vi "Measurement Logic.vi"() -> ()   [LabVIEW 2021, in "Scalar Efficiency And Load Regulation_PMIC.lvlib"]
uses:
  Scalar Efficiency And Load Regulation_PMIC.lvlib
  Measurement Configuration.ctl
  Measurement Results.ctl
  <vilib>/Plug-In SDKs/Measurements/Measure Call Context/Measure Call Context.lvclass
  <instrlib>/niDCPower/nidcpower.llb/niDCPower Sense.ctl
  <instrlib>/niDCPower/nidcpower.llb/niDCPower Source Mode.ctl
  <instrlib>/niDCPower/nidcpower.llb/niDCPower Wait For Event - Event.ctl
  <instrlib>/niDCPower/nidcpower.llb/niDCPower Output Function.ctl
  <instrlib>/niDCPower/nidcpower.llb/niDCPower Get Channel Name From String.vi
  <instrlib>/niDCPower/nidcpower.llb/niDCPower Configure Digital Edge Source Trigger With Channels.vi
  <instrlib>/niDCPower/nidcpower.llb/niDCPower Configure Digital Edge Measure Trigger With Channels.vi
panel:
  out "measure call context out":refnum<class "Measure Call Context.lvclass">
  in  "measure call context in":refnum<class "Measure Call Context.lvclass">
  out "measurement results":T1
  in  "measurement configuration":T2={"Mode of operation"=enum."Perform measurement", "DUT setup time"=1.0, "Source delay"=0.005, "Aperture time"=0.005, "Nominal output voltage"=3.3, "Source resource name"="", "Source sense"=1009, "Source current limit"=25.0, "Source maximum power"=300.0, "Load resource name"="", "Load sense"=1009, "Load voltage limit range"=6.0, "Source Voltage"=0.0, "Load Current"=0.0} {"Load sense" items=["Local"=1008, "Remote"=1009]; "Source sense" items=["Local"=1008, "Remote"=1009]}
  out "error out":errorcluster
  in  "error in":errorcluster
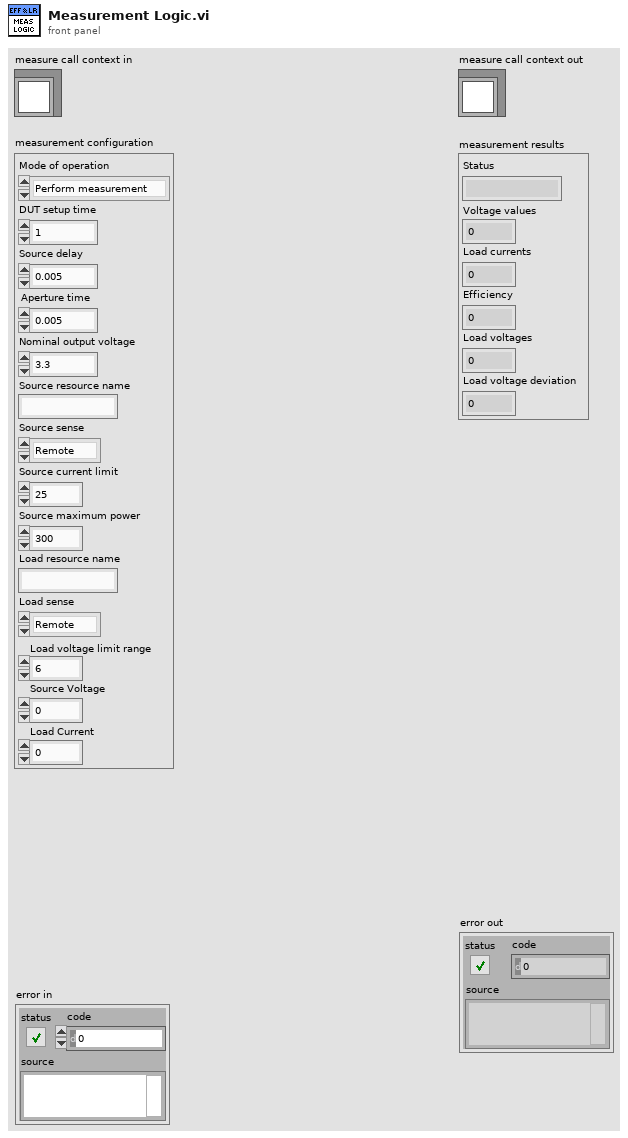
[diagram p1: front panel]
types:
  T1 = typedef "Scalar Efficiency And Load Regulation_PMIC.lvlib/Measurement Results.ctl" = cluster{"Status":string, "Voltage values":dbl, "Load currents":dbl, "Efficiency":dbl, "Load voltages":dbl, "Load voltage deviation":dbl}
  T2 = typedef "Scalar Efficiency And Load Regulation_PMIC.lvlib/Measurement Configuration.ctl" = cluster{"Mode of operation":enum32{"Power on the DUT", "Perform measurement", "Power off the DUT"}, "DUT setup time":dbl, "Source delay":dbl, "Aperture time":dbl, "Nominal output voltage":dbl, "Source resource name":string, "Source sense":i32, "Source current limit":dbl, "Source maximum power":dbl, "Load resource name":string, "Load sense":i32, "Load voltage limit range":dbl, "Source Voltage":dbl, "Load Current":dbl}
  T3 = cluster{"Voltage values":dbl, "Source out":refnum<k15>, "Source channel name":string, "Load out":refnum<k15>, "Load channel name":string, "Current values":dbl[], "Load sweep points":i32, "Source terminal name":string, "Measure terminal name":string, "Measurement Results":T1, "Source sequence name":string}
  T4 = enum32{"Power on the DUT", "Perform measurement", "Power off the DUT"}
  T5 = typedef "niDCPower Wait For Event - Event.ctl" = i32
  T6 = typedef "niDCPower Source Mode.ctl" = i32
  T7 = typedef "niDCPower Sense.ctl" = i32
  T8 = typedef "niDCPower Output Function.ctl" = i32
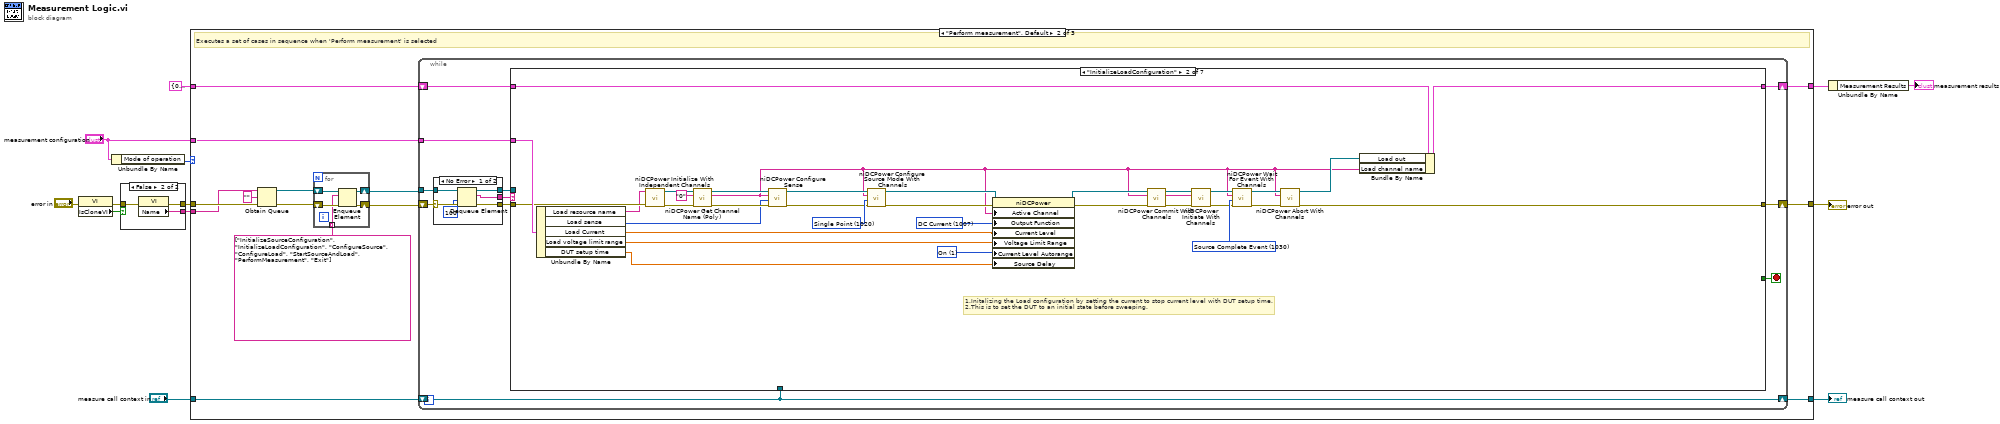
[diagram p0: block diagram]
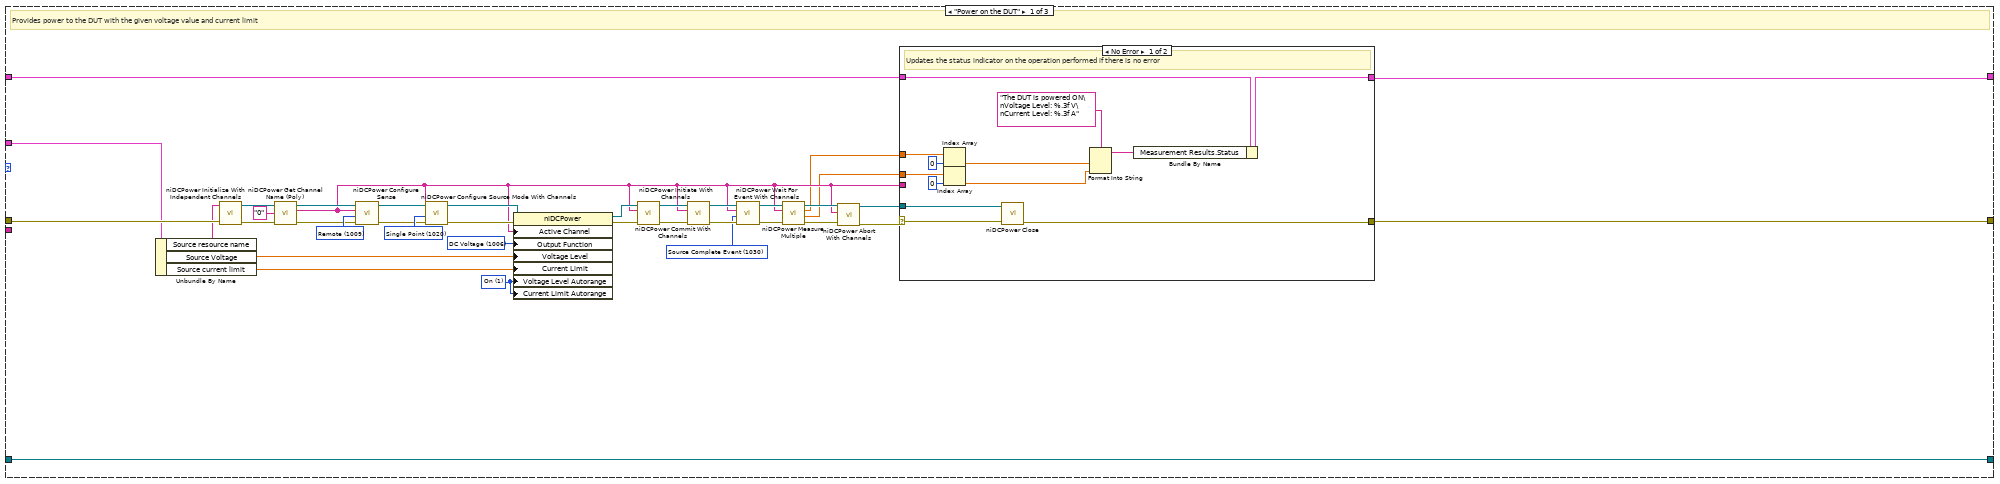
[diagram p2: hidden frame]
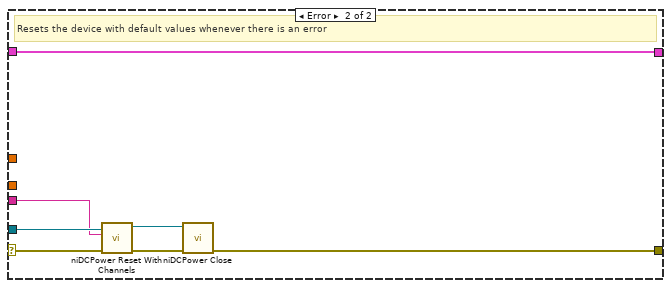
[diagram p3: hidden frame]
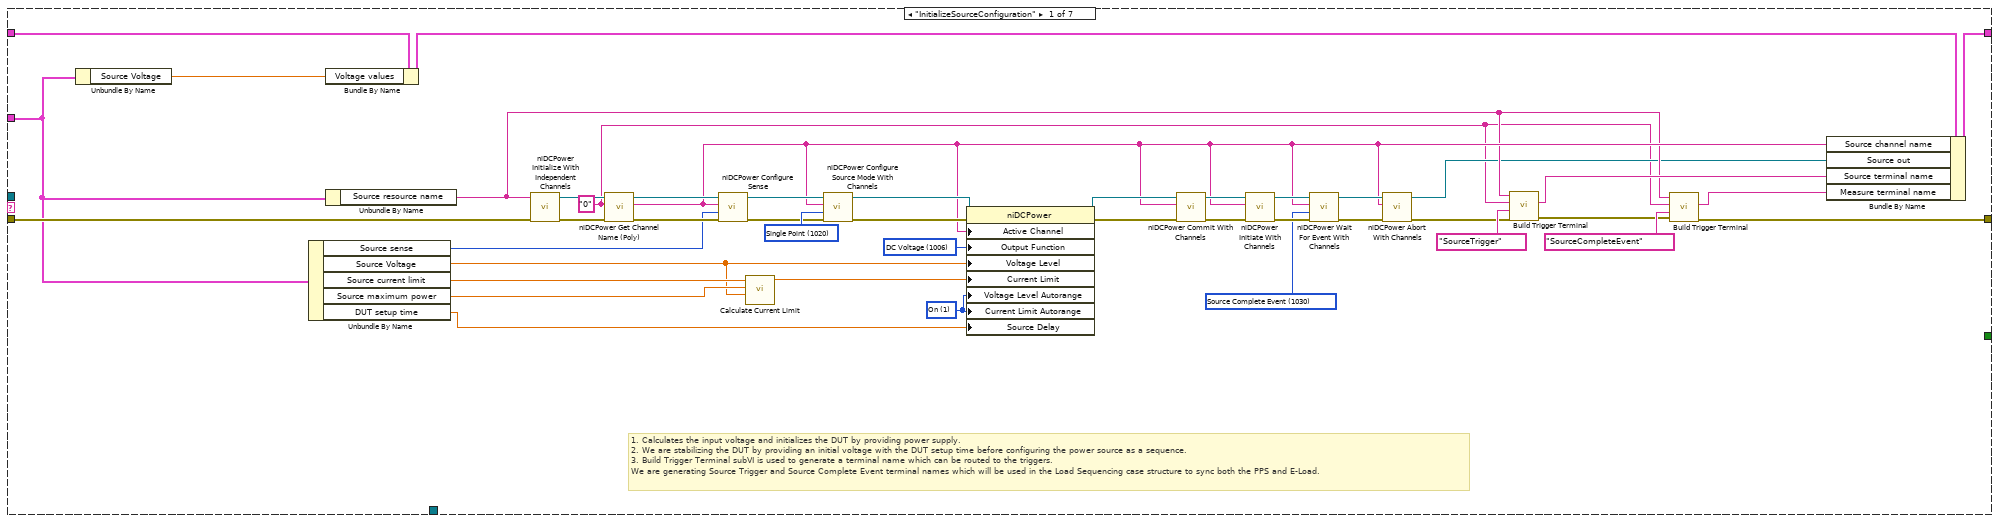
[diagram p4: hidden frame]
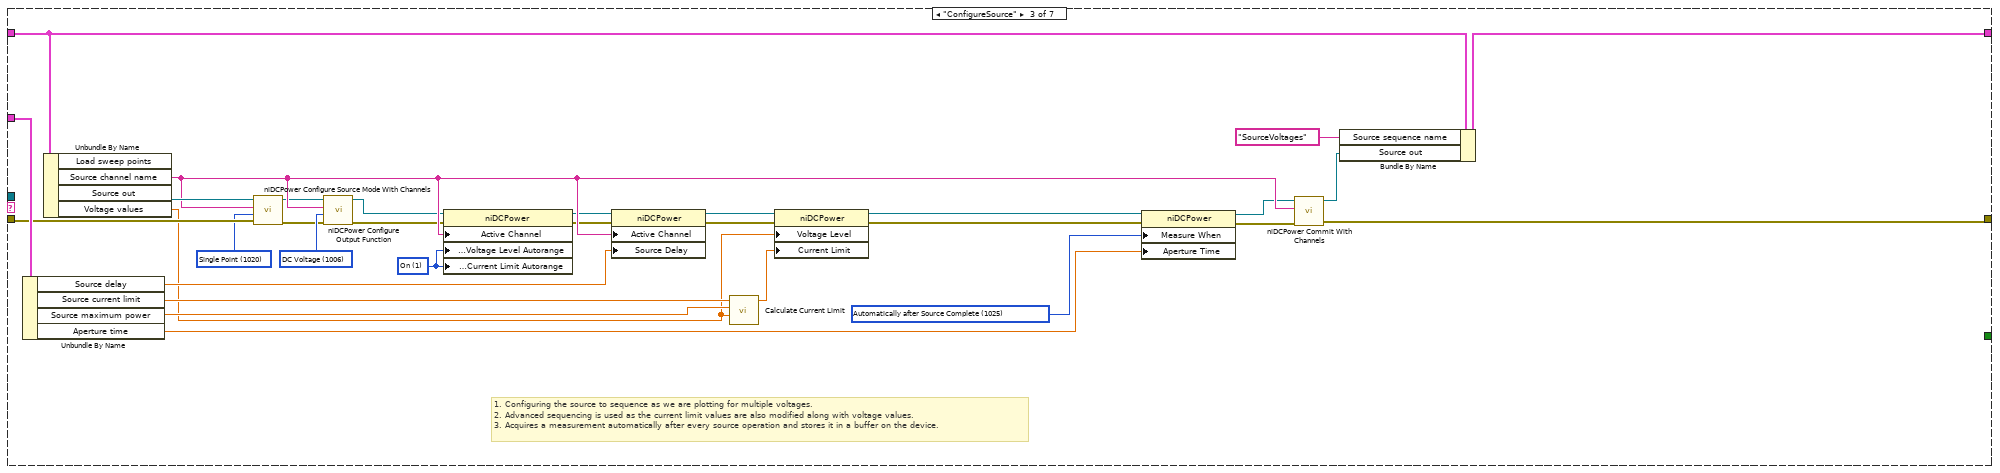
[diagram p5: hidden frame]
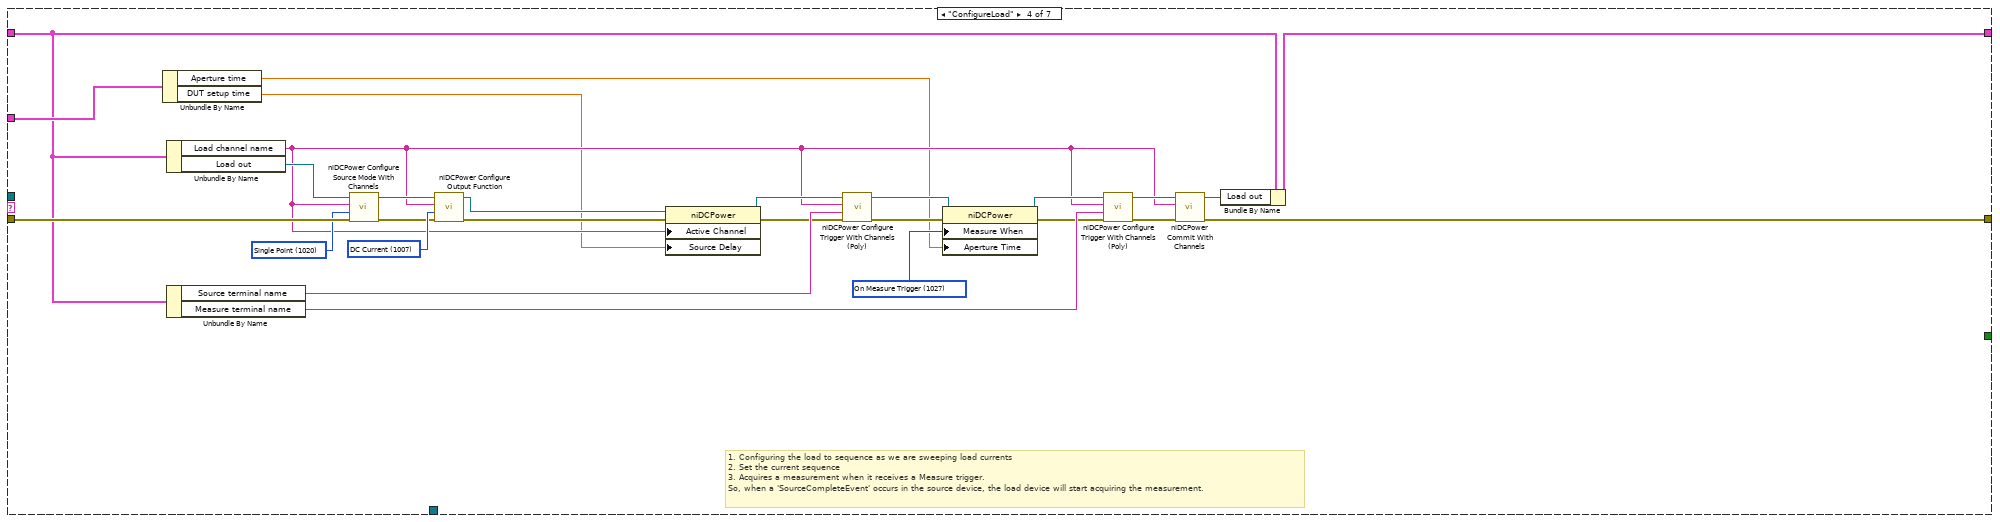
[diagram p6: hidden frame]
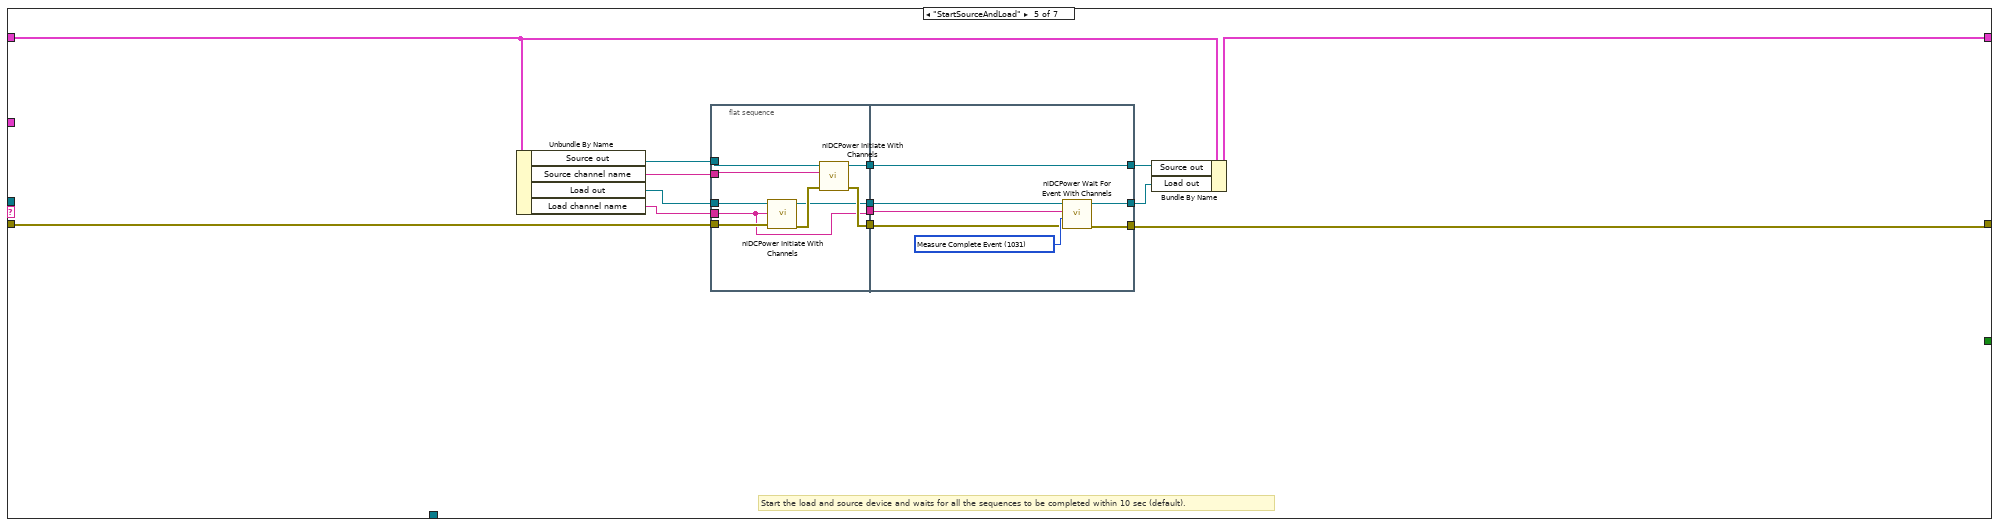
[diagram p7: hidden frame]
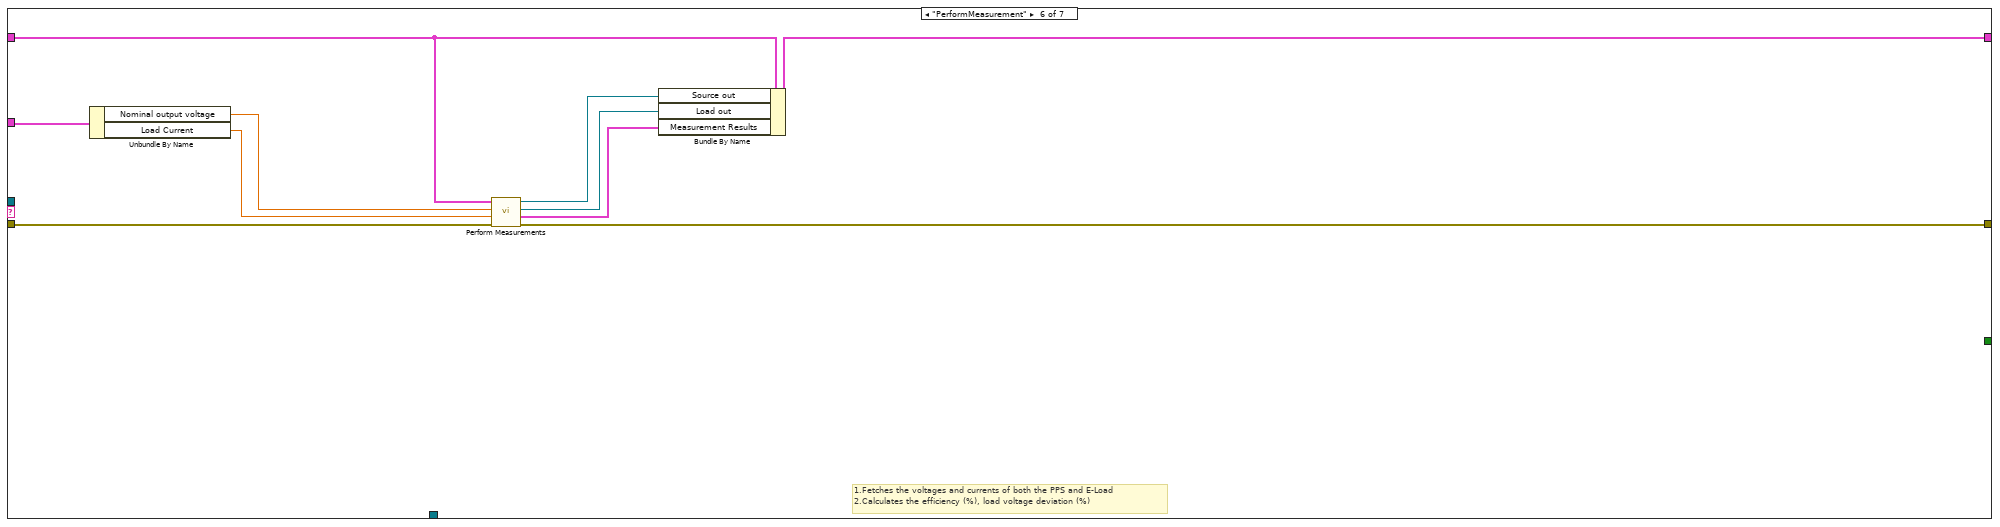
[diagram p8: hidden frame]
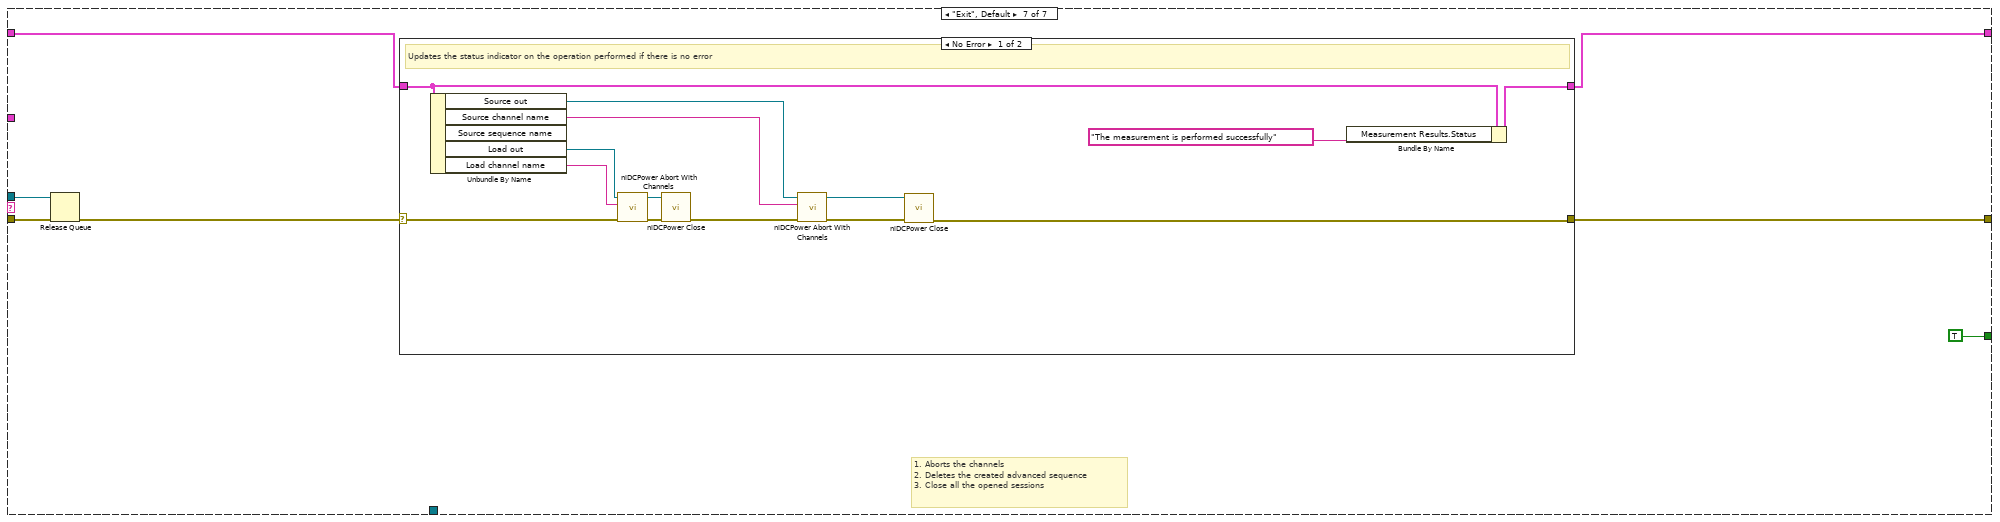
[diagram p9: hidden frame]
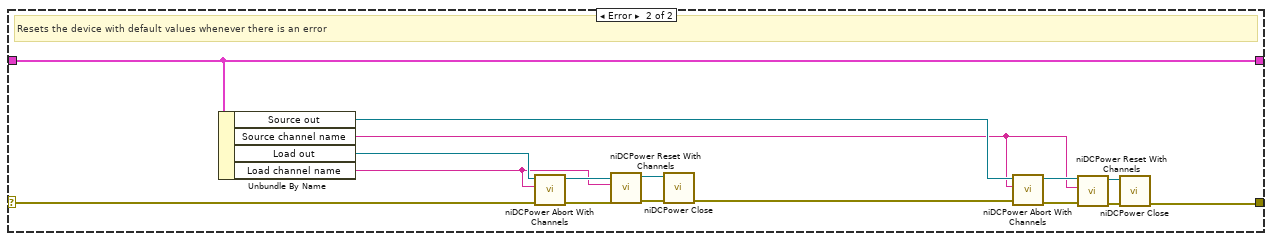
[diagram p10: hidden frame]
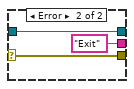
[diagram p11: hidden frame]
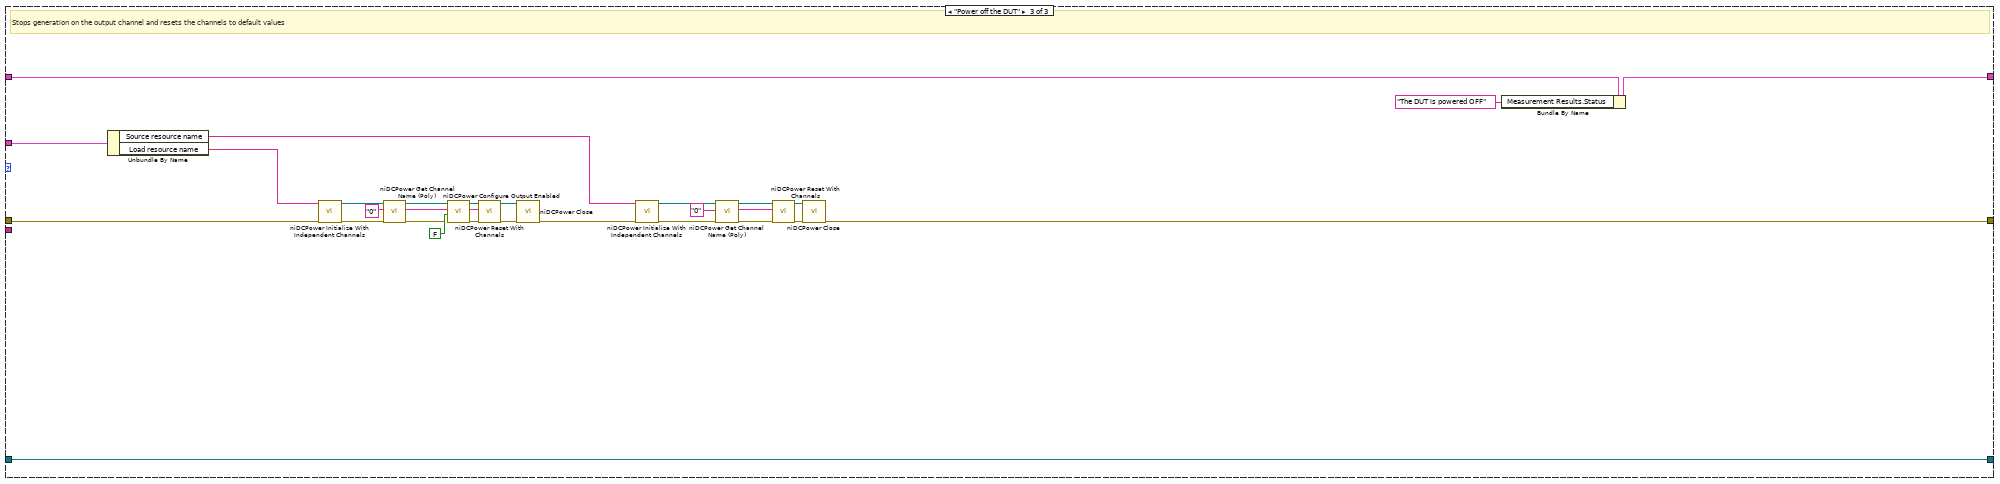
[diagram p12: hidden frame]
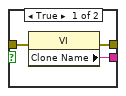
[diagram p13: hidden frame]
diagram:
  n1 = property class="VI"(error in="error in") -> (error out=w12:errorcluster, "IsCloneVI"=w13:bool)  [unwired: 1 in, 1 out]
  n2 = Unbundle By Name("measurement configuration") -> ("Mode of operation"=w5:T4)
  n3 = case shown="False" w13 {
    tunnel: [w16 w19] -> w7
    tunnel: [w15 w18] -> w6
    tunnel: w12 -> [w14 w17]
    frame True {
      n4 = property class="VI"(error in=w14) -> (error out=w16:errorcluster, "Clone Name"=w15:string)  [unwired: 1 in, 1 out]
    }
    frame False {
      n5 = property class="VI"(error in=w17) -> (error out=w19:errorcluster, "Name"=w18:string)  [unwired: 1 in, 1 out]
    }
  }
  n6 = case shown="\"Perform measurement\", Default" w5 {
    tunnel: [w21 w77 w344] -> w1
    tunnel: w7 -> [w37 w87 w343]
    tunnel: w6 -> [_ w86 _]
    tunnel: "measurement configuration" -> [w30 w83 w331]
    tunnel: [w22 w78 w327] -> w2
    tunnel: T3 {"Voltage values"=0.0, "Source out"="", "Source channel name"="", "Load out"="", "Load channel name"="", "Current values"=[], "Load sweep points"=0, "Source terminal name"="", "Measure terminal name"="", "Measurement Results"={"Status"="", "Voltage values"=0.0, "Load currents"=0.0, "Efficiency"=0.0, "Load voltages"=0.0, "Load voltage deviation"=0.0}, "Source sequence name"=""} -> [w23 w82 w329]
    tunnel: "measure call context in" -> [w20 w80 w330]
    tunnel: [w20 w79 w330] -> w3
    frame "Power on the DUT" {
      w40 = 1 items=["Off", "On"] ("Source:DC Voltage:Voltage Level Autorange")
      w41 = T5 1030 items=["Source Complete Event"=1030, "Measure Complete Event"=1031, "Sequence Iteration Complete Event"=1032, "Sequence Engine Done Event"=1033, "Pulse Complete Event"=1051, "Ready For Pulse Trigger Event"=1052] ("event")
      w52 = T6 1020 items=["Single Point"=1020, "Sequence"=1021] ("source mode")
      w47 = 1006 items=["DC Voltage"=1006, "DC Current"=1007, "Pulse Voltage"=1049, "Pulse Current"=1050] ("Source:Output Function")
      w42 = T7 1009 items=["Local"=1008, "Remote"=1009] ("sense")
      # "Provides power to the DUT with the given voltage value and current limit"
      n7 = Unbundle By Name(w30) -> ("Source resource name"=w34:string, "Source Voltage"=w29:dbl, "Source current limit"=w35:dbl)
      n8 = call <instrlib>:"niDCPower Initialize With Independent Channels.vi"("error in (no error)"=w37, "resource name"=w34) -> ("error out"=w39:errorcluster, "instrument handle out"=w43:refnum<k15>)  [unwired: 8 in]
      n9 = call-poly <instrlib>:"niDCPower Get Channel Name (Poly).vi"("index"="0", "instrument handle"=w43) -> ("name"=w26:string, "instrument handle out"=w38:refnum<k15>)  [unwired: 7 in, 1 out]
      n10 = call <instrlib>:"niDCPower Configure Sense.vi"("error in (no error)"=w39, "sense"=w42, "channel name"=w26, "instrument handle"=w38) -> ("error out"=w50:errorcluster, "instrument handle out"=w48:refnum<k15>)  [unwired: 6 in]
      n11 = call <instrlib>:"niDCPower Configure Source Mode With Channels.vi"("error in (no error)"=w50, "source mode"=w52, "channel name"=w26, "instrument handle"=w48) -> ("error out"=w51:errorcluster, "instrument handle out"=w49:refnum<k15>)  [unwired: 6 in]
      n12 = property class="niDCPower"(reference=w49, error in=w51, "Active Channel"=w26, "Output Function"=w47, "Voltage Level"=w29, "Current Limit"=w35, "Voltage Level Autorange"=w40, "Current Limit Autorange"=w40) -> (reference out=w53:refnum<k15>, error out=w54:errorcluster)
      n13 = call <instrlib>:"niDCPower Commit With Channels.vi"("error in (no error)"=w54, "channel name"=w26, "instrument handle"=w53) -> ("error out"=w56:errorcluster, "instrument handle out"=w55:refnum<k15>)  [unwired: 7 in]
      n14 = call <instrlib>:"niDCPower Initiate With Channels.vi"("error in (no error)"=w56, "channel name"=w26, "instrument handle"=w55) -> ("error out"=w44:errorcluster, "instrument handle out"=w45:refnum<k15>)  [unwired: 7 in]
      n15 = call <instrlib>:"niDCPower Wait For Event With Channels.vi"("error in (no error)"=w44, "event"=w41, "channel name"=w26, "instrument handle"=w45) -> ("error out"=w32:errorcluster, "instrument handle out"=w46:refnum<k15>)  [unwired: 6 in]
      n16 = call <instrlib>:"niDCPower Measure Multiple.vi"("error in (no error)"=w32, "channel name"=w26, "instrument handle"=w46) -> ("error out"=w31:errorcluster, "current measurements"=w24:dbl[], "voltage measurements"=w25:dbl[], "instrument handle out"=w33:refnum<k15>)  [unwired: 5 in]
      n17 = call <instrlib>:"niDCPower Abort With Channels.vi"("error in (no error)"=w31, "channel name"=w26, "instrument handle"=w33) -> ("error out"=w28:errorcluster, "instrument handle out"=w27:refnum<k15>)  [unwired: 7 in]
      n18 = case shown="No Error" w28 {
        selector: w28 -> [w69 w74]
        tunnel: [w68 w73] -> w21
        tunnel: [w67 w70] -> w22
        tunnel: w27 -> [w62 w72]
        tunnel: w26 -> [_ w71]
        tunnel: w25 -> [w61 _]
        tunnel: w24 -> [w60 _]
        tunnel: w23 -> [w59 w70]
        frame No Error {
          # "Updates the status indicator on the operation performed if there is no error"
          n19 = Index Array(array=w61, index=0) -> (element=w58:dbl)
          n20 = Index Array(array=w60, index=0) -> (element=w57:dbl)
          n21 = call <instrlib>:"niDCPower Close.vi"("error in (no error)"=w69, "instrument handle"=w62) -> ("error out"=w68:errorcluster)  [unwired: 9 out]
          n22 = Format Into String(format string="The DUT is powered ON\nVoltage Level: %.3f V\nCurrent Level: %.3f A" ("message"), w58, w57) -> (resulting string=w65:string)  [unwired: 2 in, 1 out]
          n23 = Bundle By Name(cluster=w59, "Measurement Results.Status"=w65) -> (w67:T3)
        }
        frame Error {
          # "Resets the device with default values whenever there is an error"
          n24 = call <instrlib>:"niDCPower Reset With Channels.vi"("error in (no error)"=w74, "channel name"=w71, "instrument handle"=w72) -> ("error out"=w76:errorcluster, "instrument handle out"=w75:refnum<k15>)  [unwired: 7 in]
          n25 = call <instrlib>:"niDCPower Close.vi"("error in (no error)"=w76, "instrument handle"=w75) -> ("error out"=w73:errorcluster)  [unwired: 9 out]
        }
      }
    }
    frame "Perform measurement", Default {
      # "Executes a set of cases in sequence when 'Perform measurement' is selected"
      n26 = Obtain Queue(name (unnamed)=w86, element data type="", error in (no error)=w87) -> (queue out=w89:refnum<queue>, error out=w90:errorcluster)  [unwired: 2 in, 1 out]
      n27 = for {
        shift-right: [w324] -> w84
        shift-left: w89 -> [w326]
        shift-right: [w323] -> w81
        shift-left: w90 -> [w325]
        tunnel: string[] ["InitializeSourceConfiguration", "InitializeLoadConfiguration", "ConfigureSource", "ConfigureLoad", "StartSourceAndLoad", "PerformMeasurement", "Exit"] ("Step sequence") -> [w322] mode=indexing
        n28 = Enqueue Element(queue=w326, element=w322, error in (no error)=w325) -> (queue out=w324:refnum<queue>, error out=w323:errorcluster)  [unwired: 1 in, 1 out]
      }
      n29 = while {
        tunnel: w84 -> [w101]
        tunnel: w83 -> [w97]
        shift-right: [w94] -> w78
        shift-left: w82 -> [w95]
        shift-right: [w93] -> w77
        shift-left: w81 -> [w100]
        shift-right: [w92] -> w79
        shift-left: w80 -> [w92]
        stop <- w91 stop-if-true
        n30 = case shown="No Error" w100 {
          selector: w100 -> [w316 w320]
          tunnel: w101 -> [w318 w319]
          tunnel: [w317 "Exit" ("t")] -> w99
          tunnel: [w315 w320] -> w96
          tunnel: [w313 w319] -> w98
          frame No Error {
            n31 = Dequeue Element(queue=w318, timeout in ms (-1)=100, error in (no error)=w316) -> (queue out=w313:refnum<queue>, element=w317:string, error out=w315:errorcluster)  [unwired: 1 out]
          }
          frame Error {
          }
        }
        n32 = case shown="\"InitializeLoadConfiguration\"" w99 {
          tunnel: w98 -> [_ _ _ _ _ _ w277]
          tunnel: w97 -> [w120 w177 w206 w231 _ w273 _]
          tunnel: w96 -> [w124 w176 w205 w235 w241 w275 w282]
          tunnel: w95 -> [w143 w153 w208 w228 w240 w268 w280]
          tunnel: [w144 w172 w207 w227 w237 w267 w278] -> w94
          tunnel: [w110 w175 w197 w230 w236 w274 w279] -> w93
          tunnel: w92 -> [_ _ _ _ _ _ _]
          tunnel: [_ _ _ _ _ _ TRUE] -> w91
          frame "InitializeSourceConfiguration" {
            w105 = "0" ("index")
            w126 = 1 items=["Off", "On"] ("Source:DC Voltage:Voltage Level Autorange")
            w127 = T5 1030 items=["Source Complete Event"=1030, "Measure Complete Event"=1031, "Sequence Iteration Complete Event"=1032, "Sequence Engine Done Event"=1033, "Pulse Complete Event"=1051, "Ready For Pulse Trigger Event"=1052] ("event")
            w138 = T6 1020 items=["Single Point"=1020, "Sequence"=1021] ("source mode")
            w133 = 1006 items=["DC Voltage"=1006, "DC Current"=1007, "Pulse Voltage"=1049, "Pulse Current"=1050] ("Source:Output Function")
            # "1. Calculates the input voltage and initializes the DUT by providing power supply.\n2. We are stabilizing the DUT by providing an initial voltage with the DUT setup time before configuring the power source as a sequence.\n3. Build Trigger Terminal subVI is used to generate a terminal name which can be routed to the triggers. \nWe are generating Source Trigger and Source Complete Event terminal names which will be used in the Load Sequencing case structure to sync both the PPS and E-Load."
            n33 = Unbundle By Name(w120) -> ("Source Voltage"=w102:dbl)
            n34 = Unbundle By Name(w120) -> ("Source sense"=w103:i32, "Source Voltage"=w104:dbl, "Source current limit"=w123:dbl, "Source maximum power"=w122:dbl, "DUT setup time"=w125:dbl)
            n35 = Bundle By Name(cluster=w143, "Voltage values"=w102) -> (w119:T3)
            n36 = Unbundle By Name(w120) -> ("Source resource name"=w107:string)
            n37 = call <instrlib>:"niDCPower Initialize With Independent Channels.vi"("error in (no error)"=w124, "resource name"=w107) -> ("error out"=w116:errorcluster, "instrument handle out"=w128:refnum<k15>)  [unwired: 8 in]
            n38 = call-poly <instrlib>:"niDCPower Get Channel Name (Poly).vi"("error in (no error)"=w116, "index"=w105, "instrument handle"=w128) -> ("error out"=w115:errorcluster, "name"=w117:string, "instrument handle out"=w118:refnum<k15>)  [unwired: 6 in]
            n39 = call <instrlib>:"niDCPower Configure Sense.vi"("error in (no error)"=w115, "sense"=w103, "channel name"=w117, "instrument handle"=w118) -> ("error out"=w136:errorcluster, "instrument handle out"=w134:refnum<k15>)  [unwired: 6 in]
            n40 = call "Calculate Current Limit.vi"("Voltage value"=w104, "Maximum power"=w122, "Current limit in"=w123) -> ("Current limit out"=w121:dbl)  [unwired: 8 in]
            n41 = call <instrlib>:"niDCPower Configure Source Mode With Channels.vi"("error in (no error)"=w136, "source mode"=w138, "channel name"=w117, "instrument handle"=w134) -> ("error out"=w137:errorcluster, "instrument handle out"=w135:refnum<k15>)  [unwired: 6 in]
            n42 = property class="niDCPower"(reference=w135, error in=w137, "Active Channel"=w117, "Output Function"=w133, "Voltage Level"=w104, "Current Limit"=w121, "Voltage Level Autorange"=w126, "Current Limit Autorange"=w126, "Source Delay"=w125) -> (reference out=w139:refnum<k15>, error out=w140:errorcluster)
            n43 = call <instrlib>:"niDCPower Commit With Channels.vi"("error in (no error)"=w140, "channel name"=w117, "instrument handle"=w139) -> ("error out"=w142:errorcluster, "instrument handle out"=w141:refnum<k15>)  [unwired: 7 in]
            n44 = call <instrlib>:"niDCPower Initiate With Channels.vi"("error in (no error)"=w142, "channel name"=w117, "instrument handle"=w141) -> ("error out"=w129:errorcluster, "instrument handle out"=w130:refnum<k15>)  [unwired: 7 in]
            n45 = call <instrlib>:"niDCPower Wait For Event With Channels.vi"("error in (no error)"=w129, "event"=w127, "channel name"=w117, "instrument handle"=w130) -> ("error out"=w132:errorcluster, "instrument handle out"=w131:refnum<k15>)  [unwired: 6 in]
            n46 = call <instrlib>:"niDCPower Abort With Channels.vi"("error in (no error)"=w132, "channel name"=w117, "instrument handle"=w131) -> ("error out"=w112:errorcluster, "instrument handle out"=w106:refnum<k15>)  [unwired: 7 in]
            n47 = call "Build Trigger Terminal.vi"("error in (no error)"=w112, "Trigger/Event Name"="SourceTrigger", "Channel Name"=w105, "Resource Name"=w107) -> ("error out"=w111:errorcluster, "Terminal Name"=w109:string)  [unwired: 6 in]
            n48 = call "Build Trigger Terminal.vi"("error in (no error)"=w111, "Trigger/Event Name"="SourceCompleteEvent", "Channel Name"=w105, "Resource Name"=w107) -> ("error out"=w110:errorcluster, "Terminal Name"=w108:string)  [unwired: 6 in]
            n49 = Bundle By Name(cluster=w119, "Source channel name"=w117, "Source out"=w106, "Source terminal name"=w109, "Measure terminal name"=w108) -> (w144:T3)
          }
          frame "InitializeLoadConfiguration" {
            w167 = T6 1020 items=["Single Point"=1020, "Sequence"=1021] ("source mode")
            w160 = T5 1030 items=["Source Complete Event"=1030, "Measure Complete Event"=1031, "Sequence Iteration Complete Event"=1032, "Sequence Engine Done Event"=1033, "Pulse Complete Event"=1051, "Ready For Pulse Trigger Event"=1052] ("event")
            w155 = 1 items=["Off", "On"] ("Source:DC Current:Current Level Autorange")
            w156 = 1007 items=["DC Voltage"=1006, "DC Current"=1007, "Pulse Voltage"=1049, "Pulse Current"=1050] ("Source:Output Function")
            # "1.Initalizing the Load configuration by setting the current to stop current level with DUT setup time.\n2.This is to set the DUT to an initial state before sweeping."
            n50 = Unbundle By Name(w177) -> ("Load resource name"=w147:string, "Load sense"=w146:i32, "Load Current"=w145:dbl, "Load voltage limit range"=w174:dbl, "DUT setup time"=w154:dbl)
            n51 = call <instrlib>:"niDCPower Initialize With Independent Channels.vi"("error in (no error)"=w176, "resource name"=w147) -> ("error out"=w149:errorcluster, "instrument handle out"=w157:refnum<k15>)  [unwired: 8 in]
            n52 = call-poly <instrlib>:"niDCPower Get Channel Name (Poly).vi"("error in (no error)"=w149, "index"="0", "instrument handle"=w157) -> ("error out"=w148:errorcluster, "name"=w150:string, "instrument handle out"=w152:refnum<k15>)  [unwired: 6 in]
            n53 = call <instrlib>:"niDCPower Configure Sense.vi"("error in (no error)"=w148, "sense"=w146, "channel name"=w150, "instrument handle"=w152) -> ("error out"=w164:errorcluster, "instrument handle out"=w163:refnum<k15>)  [unwired: 6 in]
            n54 = call <instrlib>:"niDCPower Configure Source Mode With Channels.vi"("error in (no error)"=w164, "source mode"=w167, "channel name"=w150, "instrument handle"=w163) -> ("error out"=w166:errorcluster, "instrument handle out"=w165:refnum<k15>)  [unwired: 6 in]
            n55 = property class="niDCPower"(reference=w165, error in=w166, "Active Channel"=w150, "Output Function"=w156, "Current Level"=w145, "Voltage Limit Range"=w174, "Current Level Autorange"=w155, "Source Delay"=w154) -> (reference out=w168:refnum<k15>, error out=w169:errorcluster)
            n56 = call <instrlib>:"niDCPower Commit With Channels.vi"("error in (no error)"=w169, "channel name"=w150, "instrument handle"=w168) -> ("error out"=w170:errorcluster, "instrument handle out"=w171:refnum<k15>)  [unwired: 7 in]
            n57 = call <instrlib>:"niDCPower Initiate With Channels.vi"("error in (no error)"=w170, "channel name"=w150, "instrument handle"=w171) -> ("error out"=w158:errorcluster, "instrument handle out"=w159:refnum<k15>)  [unwired: 7 in]
            n58 = call <instrlib>:"niDCPower Wait For Event With Channels.vi"("error in (no error)"=w158, "event"=w160, "channel name"=w150, "instrument handle"=w159) -> ("error out"=w162:errorcluster, "instrument handle out"=w161:refnum<k15>)  [unwired: 6 in]
            n59 = call <instrlib>:"niDCPower Abort With Channels.vi"("error in (no error)"=w162, "channel name"=w150, "instrument handle"=w161) -> ("error out"=w175:errorcluster, "instrument handle out"=w173:refnum<k15>)  [unwired: 7 in]
            n60 = Bundle By Name(cluster=w153, "Load out"=w173, "Load channel name"=w150) -> (w172:T3)
          }
          frame "ConfigureSource" {
            w182 = 1025 items=["Automatically after Source Complete"=1025, "On Demand"=1026, "On Measure Trigger"=1027] ("Measurement:Advanced:Measure When")
            w187 = 1 items=["Off", "On"] ("DC Voltage:Voltage Level Autorange")
            w186 = T8 1006 items=["DC Voltage"=1006, "DC Current"=1007, "Pulse Voltage"=1049, "Pulse Current"=1050] ("output function")
            w185 = T6 1020 items=["Single Point"=1020, "Sequence"=1021] ("source mode")
            # "1. Configuring the source to sequence as we are plotting for multiple voltages.\n2. Advanced sequencing is used as the current limit values are also modified along with voltage values.\n3. Acquires a measurement automatically after every source operation and stores it in a buffer on the device."
            n61 = Unbundle By Name(w206) -> ("Source delay"=w204:dbl, "Source current limit"=w203:dbl, "Source maximum power"=w202:dbl, "Aperture time"=w201:dbl)
            n62 = Unbundle By Name(w208) -> ("Source channel name"=w199:string, "Source out"=w200:refnum<k15>, "Voltage values"=w198:dbl)  [unwired: 1 out]
            n63 = call <instrlib>:"niDCPower Configure Source Mode With Channels.vi"("error in (no error)"=w205, "source mode"=w185, "channel name"=w199, "instrument handle"=w200) -> ("error out"=w183:errorcluster, "instrument handle out"=w184:refnum<k15>)  [unwired: 6 in]
            n64 = call <instrlib>:"niDCPower Configure Output Function.vi"("error in (no error)"=w183, "output function"=w186, "channel name"=w199, "instrument handle"=w184) -> ("error out"=w191:errorcluster, "instrument handle out"=w190:refnum<k15>)  [unwired: 6 out]
            n65 = property class="niDCPower"(reference=w190, error in=w191, "Active Channel"=w199, "Source:DC Voltage:Voltage Level Autorange"=w187, "Source:DC Voltage:Current Limit Autorange"=w187) -> (reference out=w188:refnum<k15>, error out=w189:errorcluster)
            n66 = property class="niDCPower"(reference=w188, error in=w189, "Active Channel"=w199, "Source Delay"=w204) -> (reference out=w194:refnum<k15>, error out=w195:errorcluster)
            n67 = call "Calculate Current Limit.vi"("Voltage value"=w198, "Maximum power"=w202, "Current limit in"=w203) -> ("Current limit out"=w178:dbl)  [unwired: 8 in]
            n68 = property class="niDCPower"(reference=w194, error in=w195, "Voltage Level"=w198, "Current Limit"=w178) -> (reference out=w192:refnum<k15>, error out=w193:errorcluster)
            n69 = property class="niDCPower"(reference=w192, error in=w193, "Measure When"=w182, "Aperture Time"=w201) -> (reference out=w180:refnum<k15>, error out=w181:errorcluster)
            n70 = call <instrlib>:"niDCPower Commit With Channels.vi"("error in (no error)"=w181, "channel name"=w199, "instrument handle"=w180) -> ("error out"=w197:errorcluster, "instrument handle out"=w179:refnum<k15>)  [unwired: 7 in]
            n71 = Bundle By Name(cluster=w208, "Source sequence name"="SourceVoltages" ("sequence name"), "Source out"=w179) -> (w207:T3)
          }
          frame "ConfigureLoad" {
            w221 = T8 1007 items=["DC Voltage"=1006, "DC Current"=1007, "Pulse Voltage"=1049, "Pulse Current"=1050] ("output function")
            w220 = 1027 items=["Automatically after Source Complete"=1025, "On Demand"=1026, "On Measure Trigger"=1027] ("Measurement:Advanced:Measure When")
            w219 = T6 1020 items=["Single Point"=1020, "Sequence"=1021] ("source mode")
            # "1. Configuring the load to sequence as we are sweeping load currents\n2. Set the current sequence\n3. Acquires a measurement when it receives a Measure trigger. \nSo, when a 'SourceCompleteEvent' occurs in the source device, the load device will start acquiring the measurement."
            n72 = Unbundle By Name(w231) -> ("Aperture time"=w209:dbl, "DUT setup time"=w210:dbl)
            n73 = Unbundle By Name(w228) -> ("Load channel name"=w211:string, "Load out"=w234:refnum<k15>)
            n74 = Unbundle By Name(w228) -> ("Source terminal name"=w233:string, "Measure terminal name"=w232:string)
            n75 = call <instrlib>:"niDCPower Configure Source Mode With Channels.vi"("error in (no error)"=w235, "source mode"=w219, "channel name"=w211, "instrument handle"=w234) -> ("error out"=w217:errorcluster, "instrument handle out"=w218:refnum<k15>)  [unwired: 6 in]
            n76 = call <instrlib>:"niDCPower Configure Output Function.vi"("error in (no error)"=w217, "output function"=w221, "channel name"=w211, "instrument handle"=w218) -> ("error out"=w213:errorcluster, "instrument handle out"=w212:refnum<k15>)  [unwired: 6 out]
            n77 = property class="niDCPower"(reference=w212, error in=w213, "Active Channel"=w211, "Source Delay"=w210) -> (reference out=w222:refnum<k15>, error out=w223:errorcluster)
            n78 = call-poly <instrlib>:"niDCPower Configure Trigger With Channels (Poly).vi"("error in (no error)"=w223, "input terminal"=w233, "channel name"=w211, "instrument handle"=w222) -> ("error out"=w214:errorcluster, "instrument handle out"=w226:refnum<k15>)  [unwired: 6 in]
            n79 = property class="niDCPower"(reference=w226, error in=w214, "Measure When"=w220, "Aperture Time"=w209) -> (reference out=w216:refnum<k15>, error out=w215:errorcluster)
            n80 = call-poly <instrlib>:"niDCPower Configure Trigger With Channels (Poly).vi"("error in (no error)"=w215, "input terminal"=w232, "channel name"=w211, "instrument handle"=w216) -> ("error out"=w224:errorcluster, "instrument handle out"=w225:refnum<k15>)  [unwired: 6 in]
            n81 = call <instrlib>:"niDCPower Commit With Channels.vi"("error in (no error)"=w224, "channel name"=w211, "instrument handle"=w225) -> ("error out"=w230:errorcluster, "instrument handle out"=w229:refnum<k15>)  [unwired: 7 in]
            n82 = Bundle By Name(cluster=w228, "Load out"=w229) -> (w227:T3)
          }
          frame "StartSourceAndLoad" {
            # "Start the load and source device and waits for all the sequences to be completed within 10 sec (default)."
            n83 = Unbundle By Name(w240) -> ("Source out"=w245:refnum<k15>, "Source channel name"=w242:string, "Load out"=w244:refnum<k15>, "Load channel name"=w243:string)
            n84 = flat-sequence {
              tunnel: [w257] -> w249
              tunnel: [w256] -> w248
              tunnel: [w255] -> w247
              tunnel: w241 -> [w254]
              tunnel: w244 -> [w253]
              tunnel: w245 -> [w252]
              tunnel: w242 -> [w251]
              tunnel: [w250] -> w246
              tunnel: w243 -> [w250]
              tunnel: w249 -> [w265]
              tunnel: w248 -> [w263]
              tunnel: w247 -> [w260]
              tunnel: [w265] -> w239
              tunnel: [w261] -> w236
              tunnel: [w262] -> w238
              tunnel: w246 -> [w259]
              frame #0 {
                n85 = call <instrlib>:"niDCPower Initiate With Channels.vi"("error in (no error)"=w254, "channel name"=w250, "instrument handle"=w253) -> ("error out"=w258:errorcluster, "instrument handle out"=w255:refnum<k15>)  [unwired: 7 in]
                n86 = call <instrlib>:"niDCPower Initiate With Channels.vi"("error in (no error)"=w258, "channel name"=w251, "instrument handle"=w252) -> ("error out"=w256:errorcluster, "instrument handle out"=w257:refnum<k15>)  [unwired: 7 in]
              }
              frame #1 {
                w264 = T5 1031 items=["Source Complete Event"=1030, "Measure Complete Event"=1031, "Sequence Iteration Complete Event"=1032, "Sequence Engine Done Event"=1033] ("event")
                n87 = call <instrlib>:"niDCPower Wait For Event With Channels.vi"("error in (no error)"=w263, "event"=w264, "channel name"=w259, "instrument handle"=w260) -> ("error out"=w261:errorcluster, "instrument handle out"=w262:refnum<k15>)  [unwired: 6 in]
              }
            }
            n88 = Bundle By Name(cluster=w240, "Source out"=w239, "Load out"=w238) -> (w237:T3)
          }
          frame "PerformMeasurement" {
            # "1.Fetches the voltages and currents of both the PPS and E-Load\n2.Calculates the efficiency (%), load voltage deviation (%)"
            n89 = Unbundle By Name(w273) -> ("Nominal output voltage"=w269:dbl, "Load Current"=w266:dbl)
            n90 = call "Perform Measurements.vi"("error in"=w275, "Load Current"=w266, "Nominal output voltage"=w269, "State data"=w268) -> ("error out"=w274:errorcluster, "Measurement Results"=w270:T1, "Load out"=w271:refnum<k15>, "Source out"=w272:refnum<k15>)  [unwired: 3 in]
            n91 = Bundle By Name(cluster=w268, "Source out"=w272, "Load out"=w271, "Measurement Results"=w270) -> (w267:T3)
          }
          frame "Exit", Default {
            # "1. Aborts the channels\n2. Deletes the created advanced sequence\n3. Close all the opened sessions"
            n92 = Release Queue(queue=w277, error in (no error)=w282) -> (error out=w281:errorcluster)  [unwired: 1 in, 2 out]
            n93 = case shown="No Error" w281 {
              selector: w281 -> [w284 w312]
              tunnel: [w283 w311] -> w279
              tunnel: w280 -> [w285 w310]
              tunnel: [w295 w310] -> w278
              frame No Error {
                # "Updates the status indicator on the operation performed if there is no error"
                n94 = Unbundle By Name(w285) -> ("Source out"=w293:refnum<k15>, "Source channel name"=w288:string, "Load out"=w292:refnum<k15>, "Load channel name"=w291:string)  [unwired: 1 out]
                n95 = call <instrlib>:"niDCPower Abort With Channels.vi"("error in (no error)"=w284, "channel name"=w291, "instrument handle"=w292) -> ("error out"=w294:errorcluster, "instrument handle out"=w286:refnum<k15>)  [unwired: 7 in]
                n96 = call <instrlib>:"niDCPower Close.vi"("error in (no error)"=w294, "instrument handle"=w286) -> ("error out"=w287:errorcluster)  [unwired: 9 in]
                n97 = call <instrlib>:"niDCPower Abort With Channels.vi"("error in (no error)"=w287, "channel name"=w288, "instrument handle"=w293) -> ("error out"=w290:errorcluster, "instrument handle out"=w289:refnum<k15>)  [unwired: 7 in]
                n98 = call <instrlib>:"niDCPower Close.vi"("error in (no error)"=w290, "instrument handle"=w289) -> ("error out"=w283:errorcluster)  [unwired: 9 in]
                n99 = Bundle By Name(cluster=w285, "Measurement Results.Status"="The measurement is performed successfully" ("message")) -> (w295:T3)
              }
              frame Error {
                # "Resets the device with default values whenever there is an error"
                n100 = Unbundle By Name(w310) -> ("Source out"=w301:refnum<k15>, "Source channel name"=w299:string, "Load out"=w298:refnum<k15>, "Load channel name"=w297:string)
                n101 = call <instrlib>:"niDCPower Abort With Channels.vi"("error in (no error)"=w312, "channel name"=w297, "instrument handle"=w298) -> ("error out"=w305:errorcluster, "instrument handle out"=w302:refnum<k15>)  [unwired: 7 in]
                n102 = call <instrlib>:"niDCPower Reset With Channels.vi"("error in (no error)"=w305, "channel name"=w297, "instrument handle"=w302) -> ("error out"=w306:errorcluster, "instrument handle out"=w307:refnum<k15>)  [unwired: 7 in]
                n103 = call <instrlib>:"niDCPower Close.vi"("error in (no error)"=w306, "instrument handle"=w307) -> ("error out"=w300:errorcluster)  [unwired: 9 out]
                n104 = call <instrlib>:"niDCPower Abort With Channels.vi"("error in (no error)"=w300, "channel name"=w299, "instrument handle"=w301) -> ("error out"=w303:errorcluster, "instrument handle out"=w304:refnum<k15>)  [unwired: 7 in]
                n105 = call <instrlib>:"niDCPower Reset With Channels.vi"("error in (no error)"=w303, "channel name"=w299, "instrument handle"=w304) -> ("error out"=w309:errorcluster, "instrument handle out"=w308:refnum<k15>)  [unwired: 7 in]
                n106 = call <instrlib>:"niDCPower Close.vi"("error in (no error)"=w309, "instrument handle"=w308) -> ("error out"=w311:errorcluster)  [unwired: 9 out]
              }
            }
          }
        }
      }
    }
    frame "Power off the DUT" {
      # "Stops generation on the output channel and resets the channels to default values"
      n107 = Unbundle By Name(w331) -> ("Source resource name"=w333:string, "Load resource name"=w336:string)
      n108 = call <instrlib>:"niDCPower Initialize With Independent Channels.vi"("error in (no error)"=w343, "resource name"=w336) -> ("error out"=w337:errorcluster, "instrument handle out"=w335:refnum<k15>)  [unwired: 8 in]
      n109 = call-poly <instrlib>:"niDCPower Get Channel Name (Poly).vi"("error in (no error)"=w337, "index"="0", "instrument handle"=w335) -> ("error out"=w348:errorcluster, "name"=w345:string, "instrument handle out"=w346:refnum<k15>)  [unwired: 6 in]
      n110 = call <instrlib>:"niDCPower Configure Output Enabled.vi"("error in (no error)"=w348, "output enabled"=FALSE, "channel name"=w345, "instrument handle"=w346) -> ("error out"=w355:errorcluster, "instrument handle out"=w354:refnum<k15>)  [unwired: 6 in]
      n111 = call <instrlib>:"niDCPower Reset With Channels.vi"("error in (no error)"=w355, "channel name"=w345, "instrument handle"=w354) -> ("error out"=w349:errorcluster, "instrument handle out"=w350:refnum<k15>)  [unwired: 7 in]
      n112 = call <instrlib>:"niDCPower Close.vi"("error in (no error)"=w349, "instrument handle"=w350) -> ("error out"=w340:errorcluster)  [unwired: 9 out]
      n113 = call <instrlib>:"niDCPower Initialize With Independent Channels.vi"("error in (no error)"=w340, "resource name"=w333) -> ("error out"=w334:errorcluster, "instrument handle out"=w332:refnum<k15>)  [unwired: 8 in]
      n114 = call-poly <instrlib>:"niDCPower Get Channel Name (Poly).vi"("error in (no error)"=w334, "index"="0", "instrument handle"=w332) -> ("error out"=w339:errorcluster, "name"=w338:string, "instrument handle out"=w341:refnum<k15>)  [unwired: 6 in]
      n115 = call <instrlib>:"niDCPower Reset With Channels.vi"("error in (no error)"=w339, "channel name"=w338, "instrument handle"=w341) -> ("error out"=w352:errorcluster, "instrument handle out"=w351:refnum<k15>)  [unwired: 7 in]
      n116 = call <instrlib>:"niDCPower Close.vi"("error in (no error)"=w352, "instrument handle"=w351) -> ("error out"=w344:errorcluster)  [unwired: 9 out]
      n117 = Bundle By Name(cluster=w329, "Measurement Results.Status"="The DUT is powered OFF") -> (w327:T3)
    }
  }
  "error out" <- w1
  "measure call context out" <- w3
  n118 = Unbundle By Name(w2) -> ("Measurement Results"=→"measurement results":T1)
